vi "SimpleDigitizer_VI.vi"() -> ()   [LabVIEW 2014]
uses:
  <vilib>/rvi/Emulation/niFpgaGetClockAttributes.vi
  <vilib>/rvi/Emulation/niFpgaSctlEmulationGetInTimedLoop.vi
  <vilib>/rvi/Emulation/niFpgaEmulationReportErrorSimple.vi
  <vilib>/rvi/eio/common/nirviEmuTemplateMethod_errors.vi
  <vilib>/rvi/Emulation/niFpgaCriticalErrorInLSC.vi
  <vilib>/rvi/interface/RandomDataEmulation/niFpgaRandomDataHandleErrors.vi
  <vilib>/rvi/FXPMathLib/FxpInterpret/XNode/nifxpmath_Interpret.xnode
  <vilib>/eio/EIONode/EIONode.xnode
  <vilib>/rvi/DataTransferAndStorage/Container/XNode/niFpgaContainer.xnode
  <vilib>/rvi/interface/RandomDataEmulation/nirviRandomDataFpgaReadWriteTemplate.vi
  <instrlib>/_niInstr/Basic Elements/v1/FPGA/niInstr Basic Elements v1 FPGA.lvlib
panel:
  in  "Trigger":bool
  out "Analog In":i32
  out "Analog Out":i16
  out "sampleCt":i32
  in  "Trigger Out":bool
  in  "Acquire":bool
  in  "Number of Samples":u32
  in  "Sample Interval (uSec)":u32
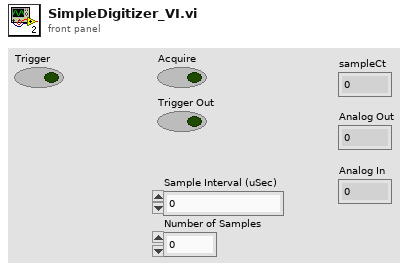
[diagram p1: front panel]
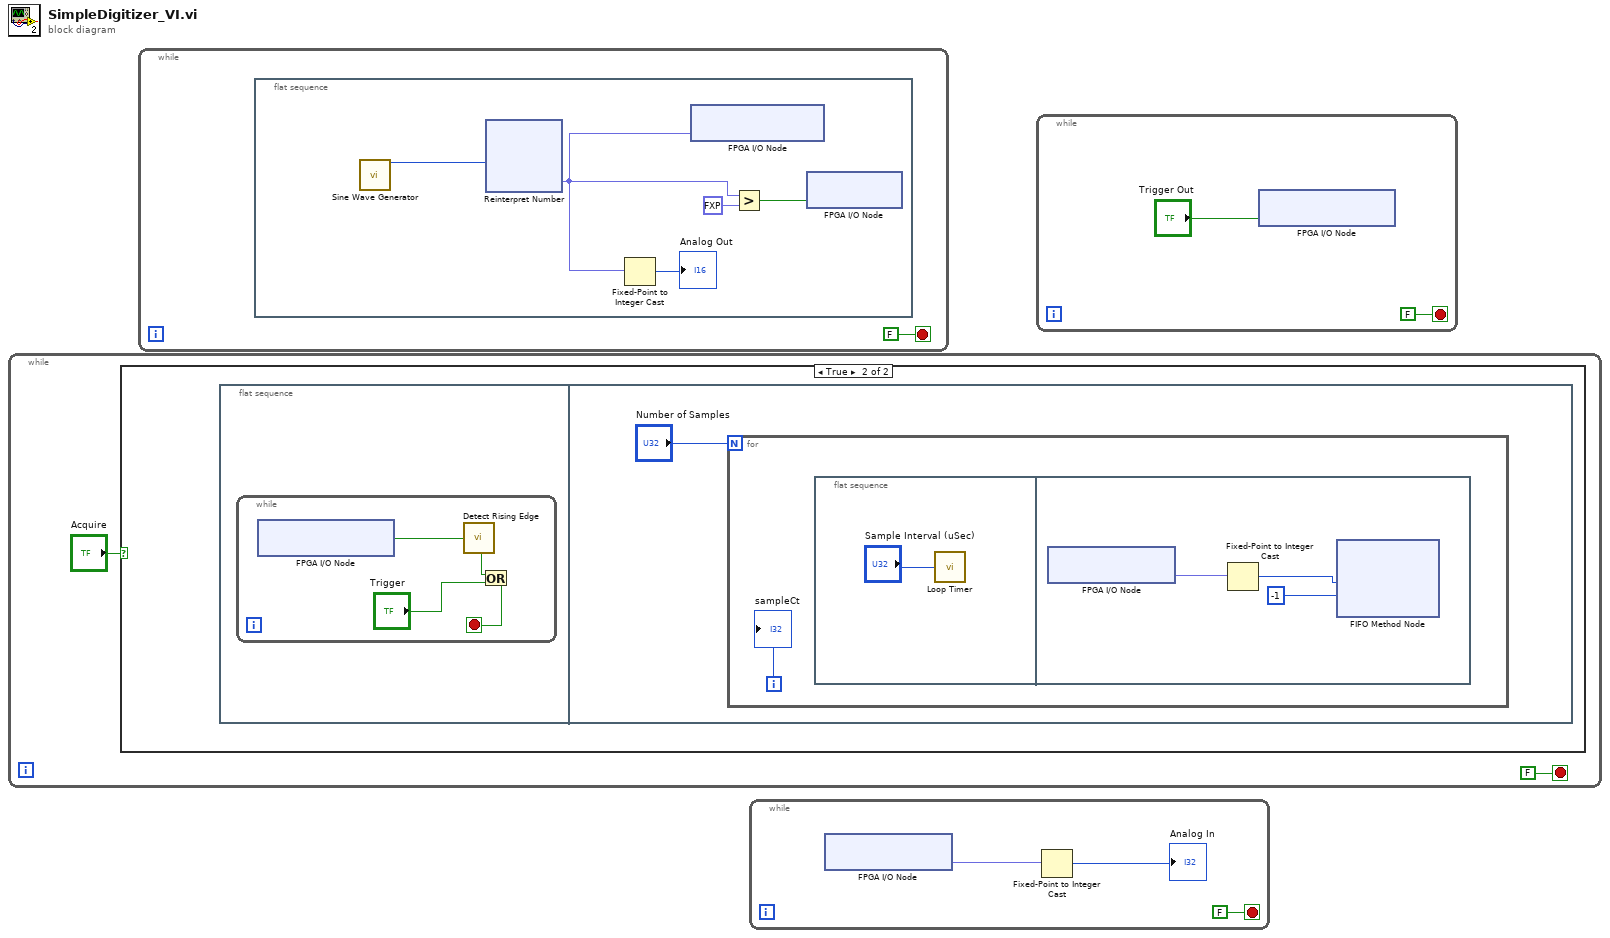
[diagram p0: block diagram]
diagram:
  n1 = while {
    stop <- FALSE stop-if-true
    n2 = case shown="True" "Acquire" {
      frame False {
      }
      frame True {
        n3 = flat-sequence {
          frame #0 {
            n4 = while {
              stop <- w4 stop-if-true
              n5 = xnode "FPGA I/O Node"() -> ("Connector1/DIO0"=w6:bool)  [unwired: 1 in, 1 out]
              n6 = call <instrlib>:"Detect Rising Edge.vi"("signal"=w6) -> ("edge detected"=w5:bool)  [unwired: 14 in]
              n7 = Or(x=w5, y="Trigger") -> (x .or. y?=w4:bool)
            }
          }
          frame #1 {
            n8 = for {
              N: "Number of Samples" -> [_]
              i -> [w8]
              n9 = flat-sequence {
                frame #0 {
                  n10 = call "Loop Timer"("Count(uSec)"="Sample Interval (uSec)") -> ()  [unwired: 1 out]
                }
                frame #1 {
                  n11 = xnode "FPGA I/O Node"() -> ("Connector1/AI0"=w11:fxp<+/-,27,5>)  [unwired: 1 in, 1 out]
                  n12 = Fixed-Point to Integer Cast(1:w11) -> (0:w10:i32)
                  n13 = xnode ("FIFO Method Node")("Element"=w10, "Timeout"=-1) -> ()  [unwired: 1 in, 2 out]
                }
              }
              "sampleCt" <- w8
            }
          }
        }
      }
    }
  }
  n14 = while {
    stop <- FALSE stop-if-true
    n15 = flat-sequence {
      frame #0 {
        n16 = call "Sine Wave Generator"() -> ("sine out"=w16:i16)  [unwired: 15 in]
        n17 = xnode "Reinterpret Number"("x"=w16) -> ("y"=w15:fxp<+/-,16,3>)
        n18 = Fixed-Point to Integer Cast(1:w15) -> (0:→"Analog Out":i16)
        n19 = xnode "FPGA I/O Node"("Connector1/AO0"=w15) -> ()  [unwired: 1 in, 1 out]
        n20 = Greater?(x=w15, y=fxp<+/-,16,1> 0.0) -> (0:w18:bool)
        n21 = xnode "FPGA I/O Node"("User LED1"=w18) -> ()  [unwired: 1 in, 1 out]
      }
    }
  }
  n22 = while {
    stop <- FALSE stop-if-true
    n23 = xnode "FPGA I/O Node"() -> ("Connector1/AI0"=w21:fxp<+/-,27,5>)  [unwired: 1 in, 1 out]
    n24 = Fixed-Point to Integer Cast(1:w21) -> (0:→"Analog In":i32)
  }
  n25 = while {
    stop <- FALSE stop-if-true
    n26 = xnode "FPGA I/O Node"("Connector1/DIO1"="Trigger Out") -> ()  [unwired: 1 in, 1 out]
  }
